vi "Write Polling Iterations.vi"(8 "error in (no error)":errorcluster, 10 "Polling Iterations":u32, 11 "CS++BaseActor in":refnum<class "CS++BaseActor.lvclass">) -> (0 "error out":errorcluster, 3 "CS++BaseActor out":refnum<class "CS++BaseActor.lvclass">)   [LabVIEW 2016, in "CS++BaseActor.lvlib" / "CS++BaseActor.lvclass"]
doc: "Write number of requested polling iteration to attribute."
uses:
  CS++BaseActor.lvclass
  Classes/CS++ProcessVariables/ProcessVariable/PV.lvclass
  CS++BaseActor.lvclass/CS++BaseActor.ctl
  Classes/CS++ProcessVariables/ProcessVariable/PV.lvclass/PV.ctl
  Classes/CS++ProcessVariables/ProcessVariable/Write Timestamp.vi
  Classes/CS++ProcessVariables/ProcessVariable/Write Data.vi
  Classes/CS++ProcessVariables/PVConnection/PVConnection.lvclass
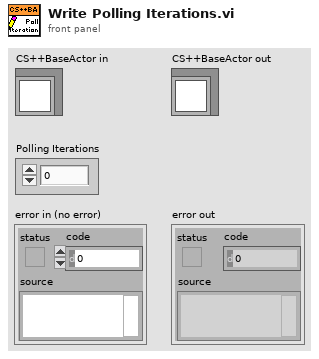
[diagram p1: front panel]
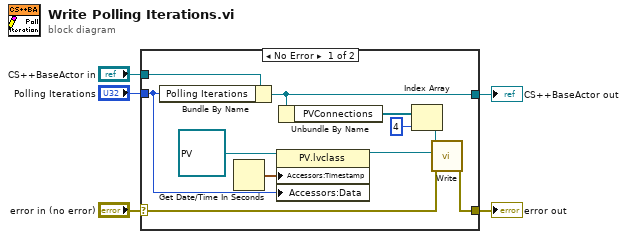
[diagram p0: block diagram]
diagram:
  n1 = case shown="No Error" "error in (no error)" {
    selector: "error in (no error)" -> [w7 w17]
    tunnel: [w6 w17] -> w4
    tunnel: [w15 w18] -> w2
    tunnel: "CS++BaseActor in" -> [w16 w18]
    tunnel: "Polling Iterations" -> [w12 _]
    frame No Error {
      n2 = Bundle By Name(cluster=w16, "Polling Iterations"=w12) -> (w15:refnum<class "CS++BaseActor.lvclass">)
      n3 = Get Date/Time In Seconds() -> (seconds since 1Jan1904=w14:timestamp)
      n4 = property class="PV.lvclass"(reference=refnum<class "PV.lvclass"> refnum ("CS++ProcessVariables.lvlib:PV.lvclass"), "Accessors:Timestamp"=w14, "Accessors:Data"=w12) -> (reference out=w8:refnum<class "PV.lvclass">)  [unwired: 1 in, 1 out]
      n5 = Unbundle By Name(w15) -> ("PVConnections"=w10:refnum<class "PVConnection.lvclass">[])
      n6 = Index Array(array=w10, index=4) -> (element=w9:refnum<class "PVConnection.lvclass">)
      n7 = call "Write.vi"("error in (no error)"=w7, "PV"=w8, "PVConnection in"=w9) -> ("error out"=w6:errorcluster)  [unwired: 7 in, 1 out]
    }
    frame Error {
    }
  }
  "error out" <- w4
  "CS++BaseActor out" <- w2
